vi "analyze memory usage.vi"(8 "error in (no error)":errorcluster, 10 "offset (0)":i64, 11 "file path":path) -> (0 "error out":errorcluster, 2 "memory stats":T1, 3 "data":dbl[](array[numeric]))   [LabVIEW 2014]
uses:
  <vilib>/gmath/statdist.llb/st_Percentiles (scalar).vi
  <vilib>/Analysis/NI_AALBase.lvlib
  <vilib>/gmath/NI_Gmath.lvlib
  <vilib>/Analysis/NI_AALPro.lvlib
panel:
  out "free memory":dbl[](graph)
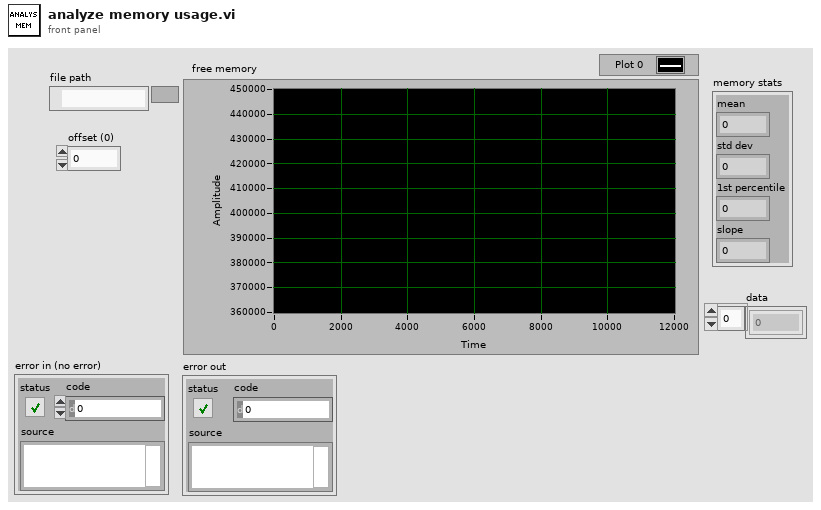
[diagram p1: front panel]
types:
  T1 = cluster{"mean":dbl, "std dev":dbl, "1st percentile":dbl, "slope":dbl}
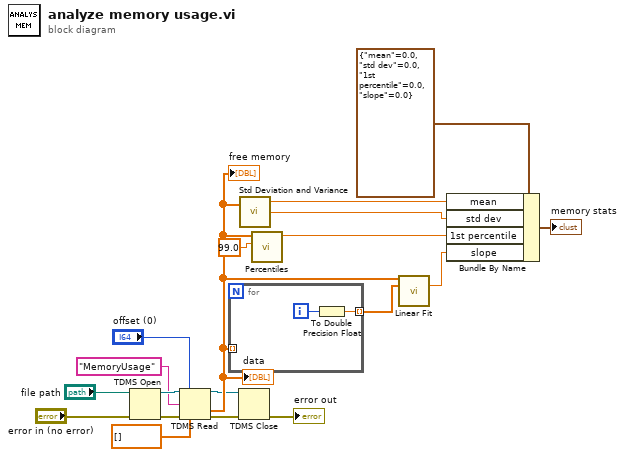
[diagram p0: block diagram]
diagram:
  n1 = TDMS Open(8:"error in (no error)", 11:"file path") -> (0:w14:errorcluster, 3:w13:refnum<k34>)  [unwired: 5 in]
  n2 = TDMS Read(0:w13, 1:"offset (0)", 7:"MemoryUsage" ("channel name(s) in"), 11:w14, 12:dbl[] []) -> (4:w11:refnum<k34>, 10:w18:dbl[], 15:w10:errorcluster)  [unwired: 3 in, 3 out]
  "free memory" <- w18
  "data" <- w18
  n3 = for {
    tunnel: w18 -> [_] mode=indexing
    tunnel: [w20] -> w17 mode=indexing
    i -> [w21]
    n4 = To Double Precision Float(number=w21) -> (double precision float=w20:dbl)
  }
  n5 = TDMS Close(8:w10, 11:w11) -> (0:→"error out":errorcluster)  [unwired: 1 out]
  n6 = call <vilib>:"Std Deviation and Variance.vi"("X"=w18) -> ("mean"=w7:dbl, "standard deviation"=w6:dbl)  [unwired: 1 in, 1 out]
  n7 = call-poly <vilib>:"Percentiles.vi"("p"=99.0, "x array"=w18) -> ("percentile"=w5:dbl)  [unwired: 8 in, 1 out]
  n8 = call <vilib>:"Linear Fit.vi"("Y"=w18, "X"=w17) -> ("slope"=w4:dbl)  [unwired: 9 in, 4 out]
  n9 = Bundle By Name(cluster=T1 {"mean"=0.0, "std dev"=0.0, "1st percentile"=0.0, "slope"=0.0}, "mean"=w7, "std dev"=w6, "1st percentile"=w5, "slope"=w4) -> (→"memory stats":T1)
